vi "Main.vi"(0 "User Signal":u16 format="%.0x", 1 "Signal Operator":T1, 2 "Generate":bool, 5 "Speed Mode":T3, 7 "Target Address":u16 max=127 format="%.0x", 9 "Addressing bit":T2, 11 "Error In":errorcluster) -> (4 "Digital Waveform Graph":digitaldata(graph), 15 "Error out":errorcluster)   [LabVIEW 2020, in "I2C Controller.lvlib"]
doc: "This VI is to move from one state to other to perform ertain functionality."
uses:
  I2C Controller.lvlib
  Typedefs/Speed Control.ctl
  Typedefs/Addressing Bit.ctl
  Typedefs/Signal Operator.ctl
  Typedefs/Operator.ctl
  Typedefs/Controller Data.ctl
  Class/Parent Class/Speed Mode/Speed Mode.lvclass
  Class/Parent Class/Address/Address.lvclass
  Typedefs/User event operator.ctl
  <vilib>/numeric/Random Number (Range) U64.vi
  <vilib>/numeric/sub_Random U32.vi
panel:
  out "Read Signal":u64
  # "I2C Controller"
  # "Bit timing Parameters"
  # "Data"
  # "Generate signals"
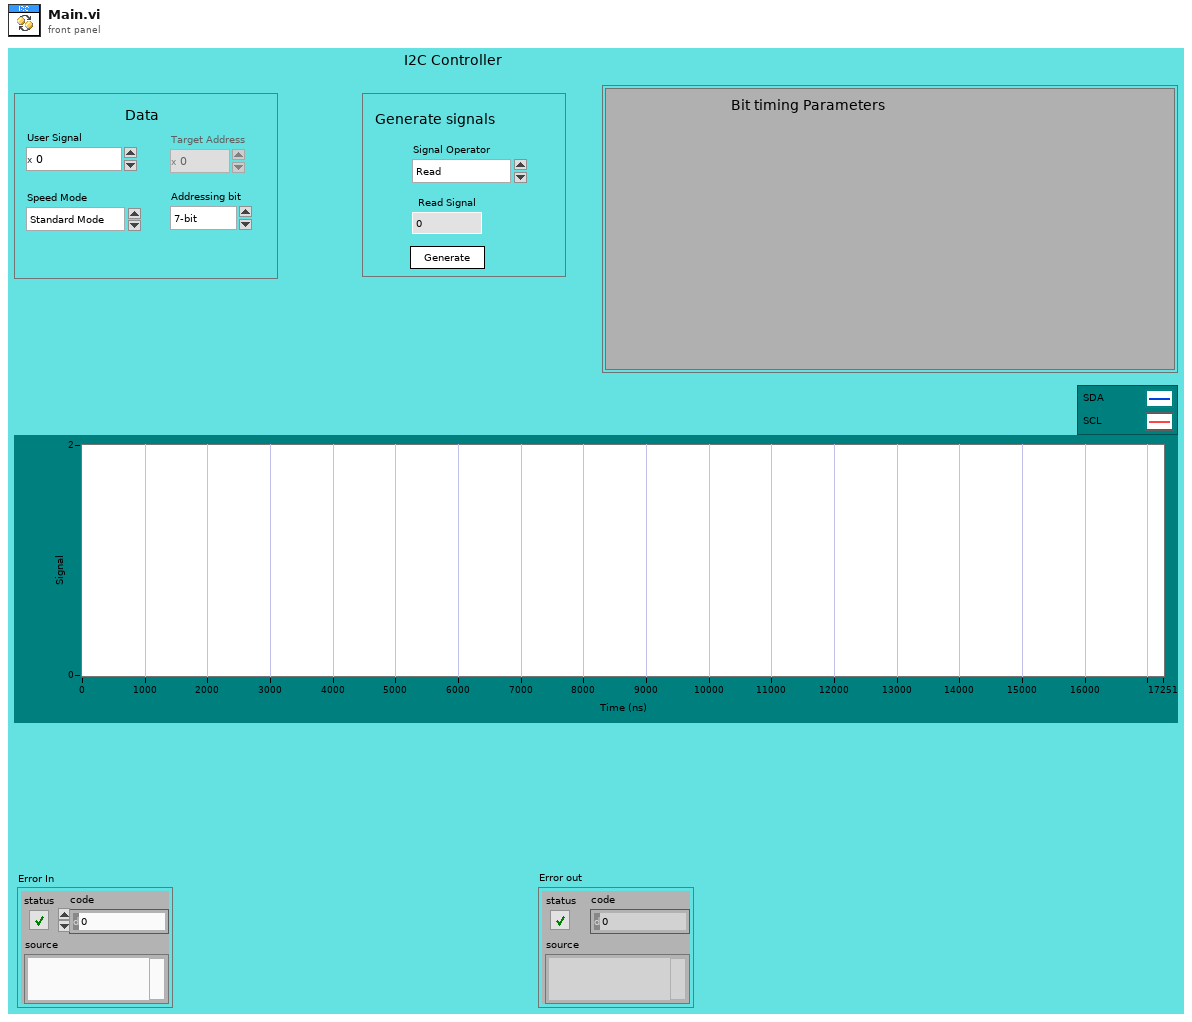
[diagram p1: front panel]
types:
  T1 = typedef "I2C Controller.lvlib/Signal Operator.ctl" = enum16{"Read", "Write", "Write-Read"}
  T2 = typedef "I2C Controller.lvlib/Addressing Bit.ctl" = enum16{"7-bit", "10-bit"}
  T3 = typedef "I2C Controller.lvlib/Speed Control.ctl" = enum16{"Standard Mode", "Fast Mode", "Fast-Plus Mode"}
  T4 = typedef "I2C Controller.lvlib/Controller Data.ctl" = cluster{"Target Address":u16, "User Signal":u8, "Read Signal":u64, "R/W Bit":i32, "Address Flag":bool, "Signal Size":i32, "Class Path":path, "Addressing bit":T2, "Speed Mode":T3, "Signal Operator":T1, "Generated Address":i16[], "User signal array":i16[], "Signal array":i16[], "Clock Signal":i16[], "Data":u8[][], "Time array":dbl[], "DVR Out":refnum<data-value>, "Addrerss DVR":refnum<data-value>, "Asynch Ref":refnum<vi>, "Digital Waveform Graph":digitaldata}
  T5 = typedef "I2C Controller.lvlib/Operator.ctl" = enum16{"Create Queue", "Enqueue", "Enstack", "Dequeue", "Flush Queue", "Release Queue"}
  T6 = typedef "I2C Controller.lvlib/User event operator.ctl" = enum16{"Create", "Generate Stop", "Destroy"}
  T7 = enum8{"Enabled", "Disabled", "Disabled and Grayed Out"}
  T8 = cluster{"Clock frequency":dbl, " T hd;sta":dbl, "T low":dbl, "T high":dbl, "T su;sta":dbl, "T hd;dat":dbl, "T su;dat":dbl, "T su;sto":dbl, "T buf":dbl}
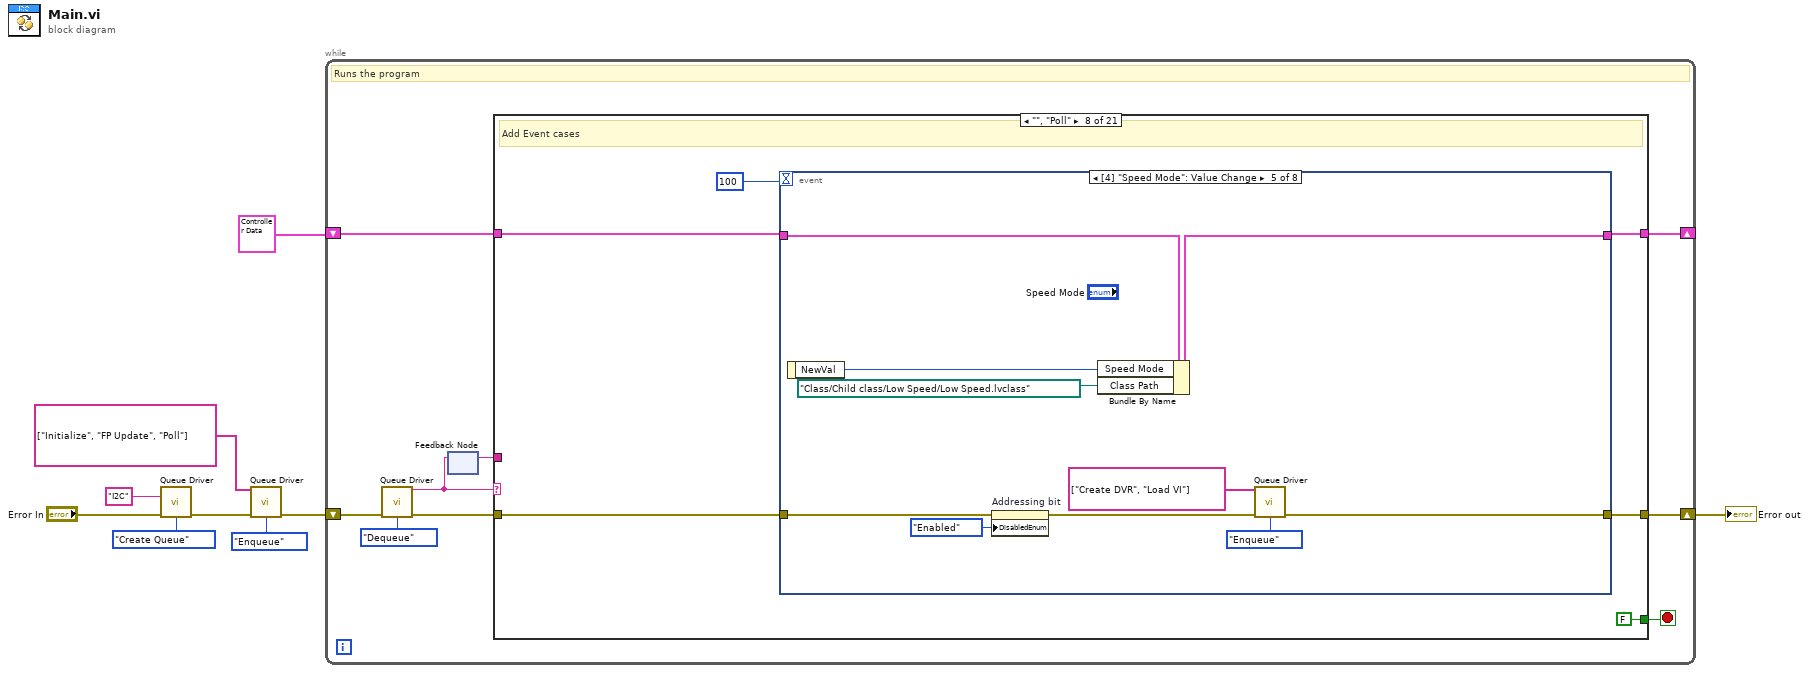
[diagram p0: block diagram]
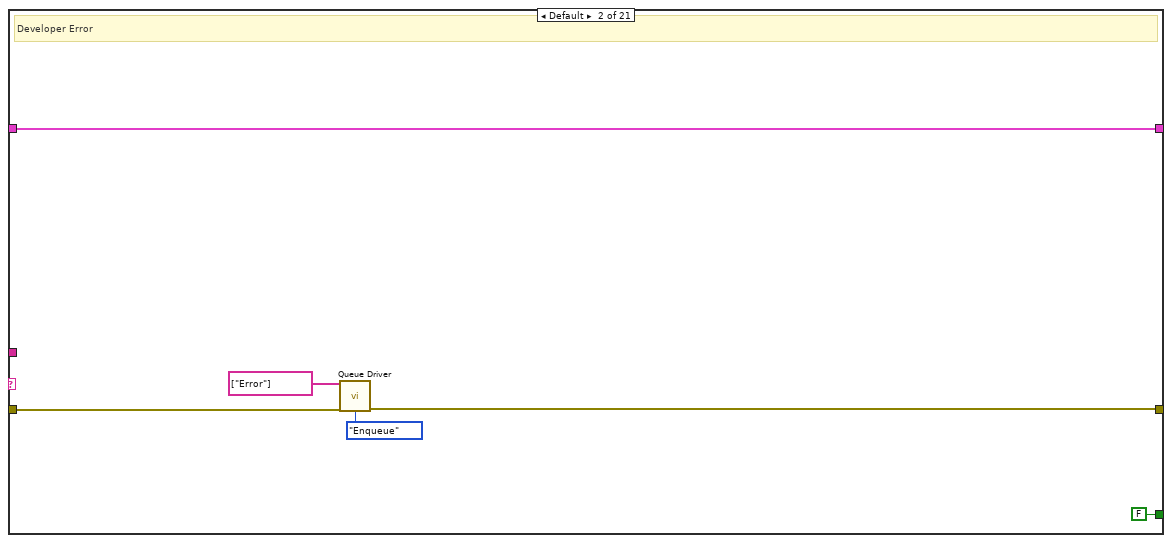
[diagram p3: hidden frame]
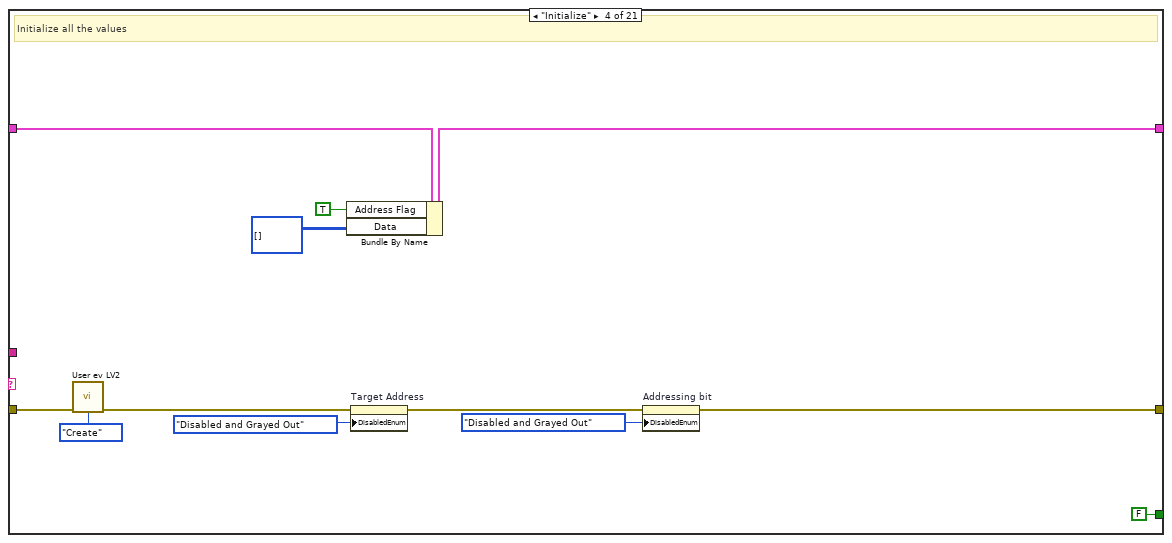
[diagram p5: hidden frame]
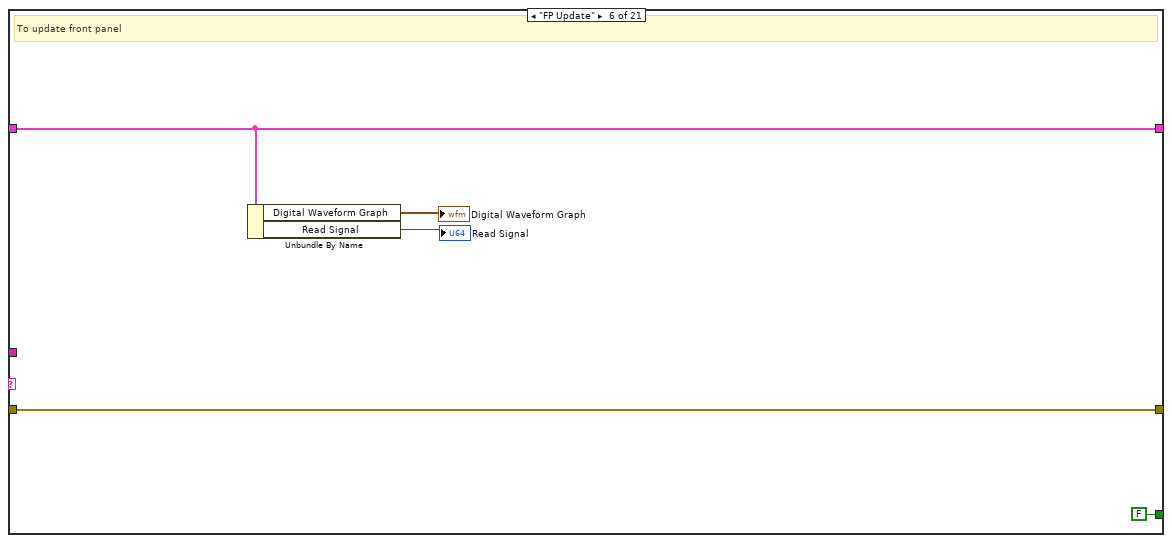
[diagram p7: hidden frame]
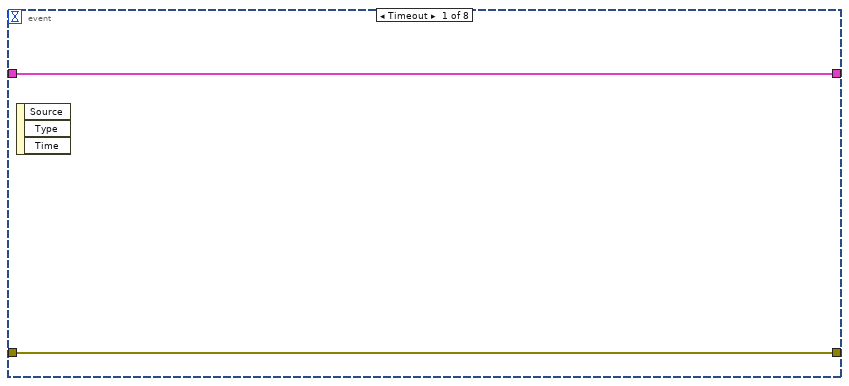
[diagram p9: hidden frame]
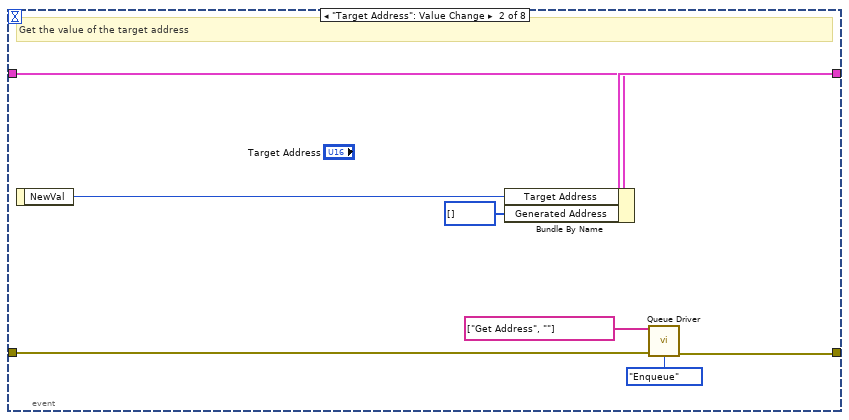
[diagram p10: hidden frame]
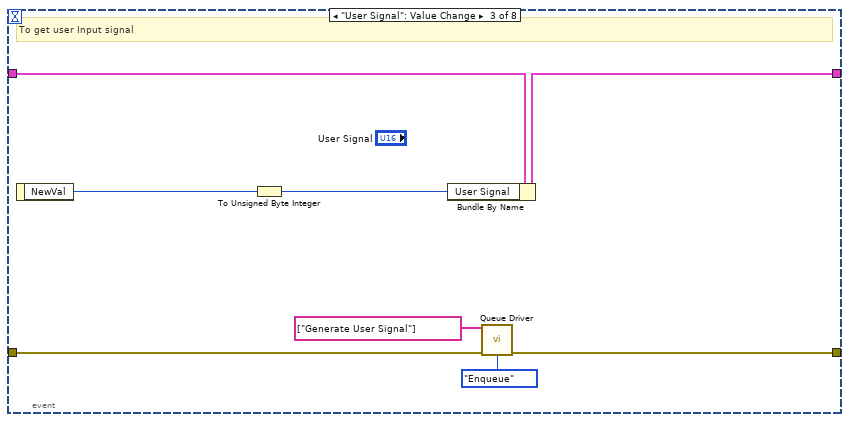
[diagram p11: hidden frame]
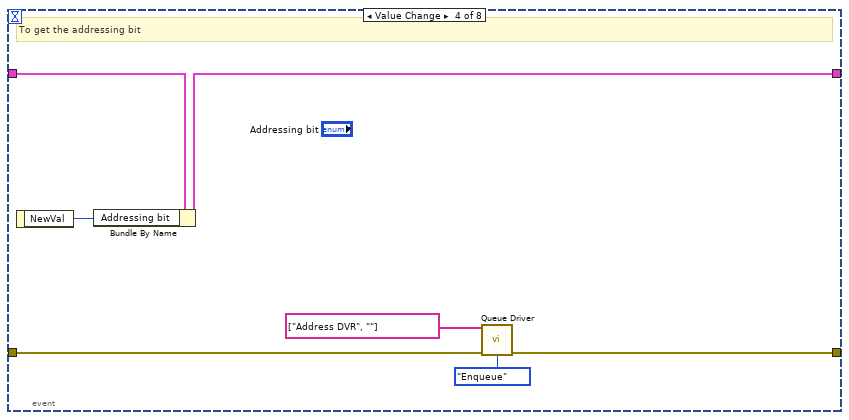
[diagram p12: hidden frame]
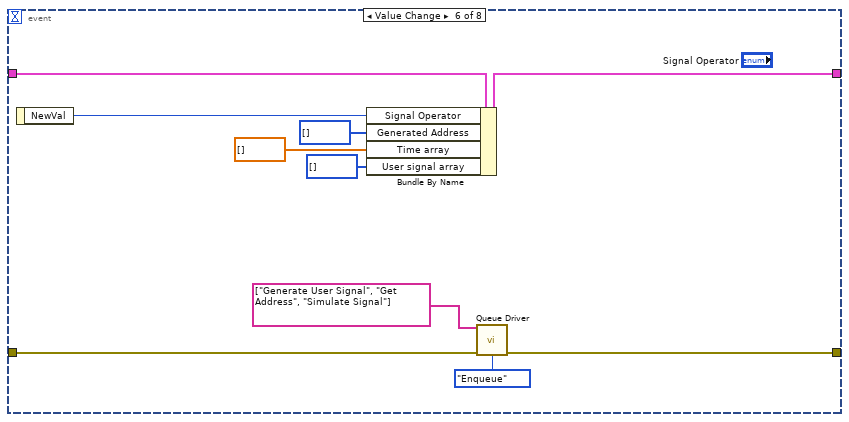
[diagram p13: hidden frame]
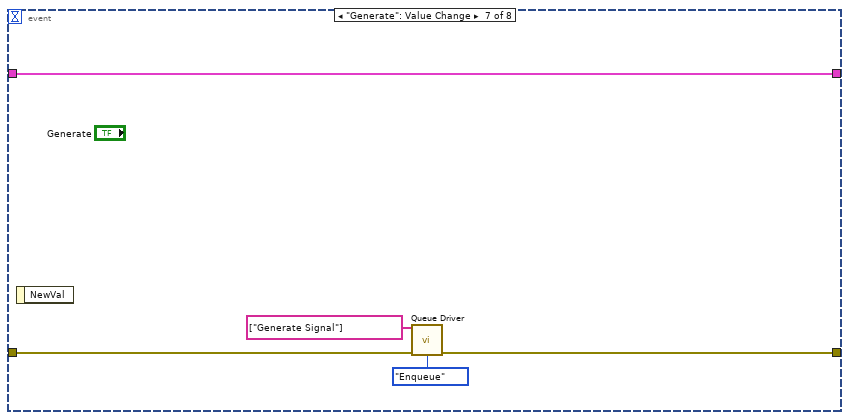
[diagram p14: hidden frame]
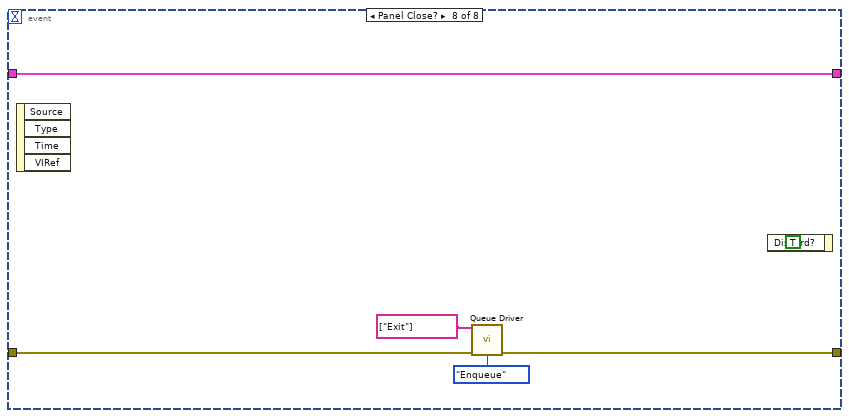
[diagram p15: hidden frame]
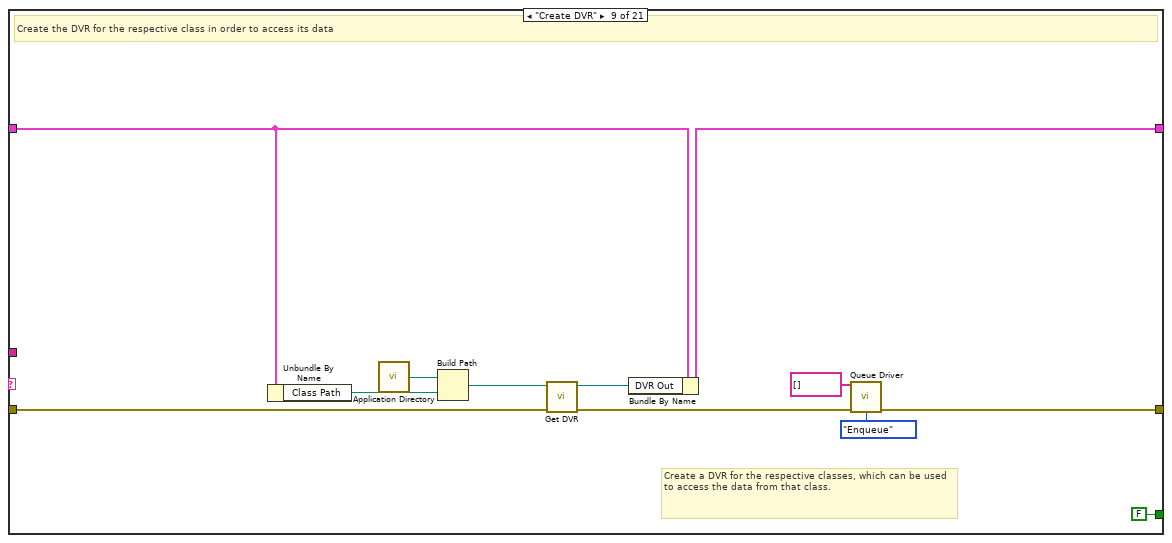
[diagram p16: hidden frame]
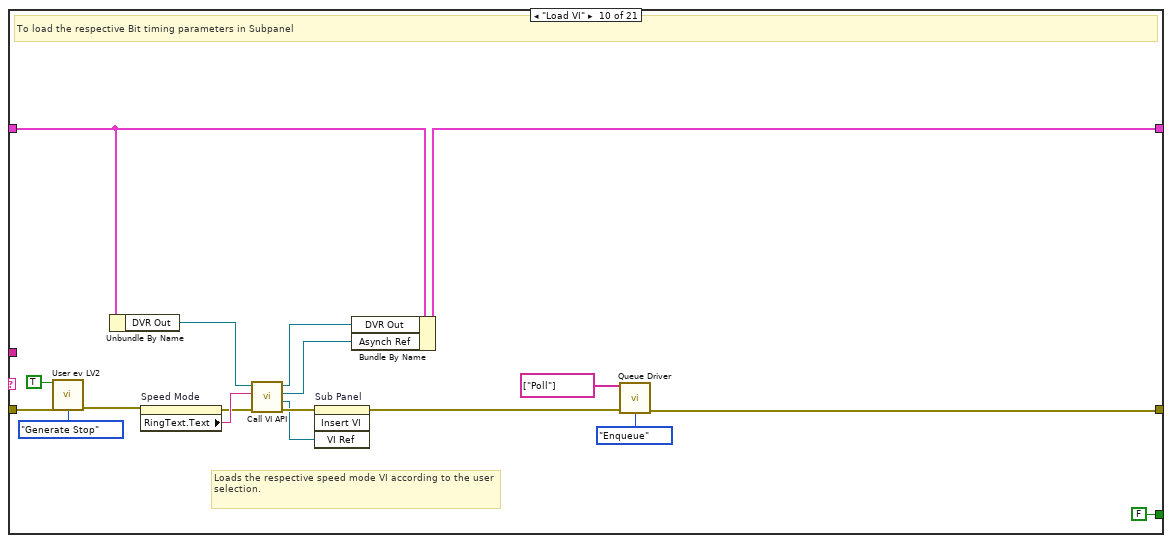
[diagram p17: hidden frame]
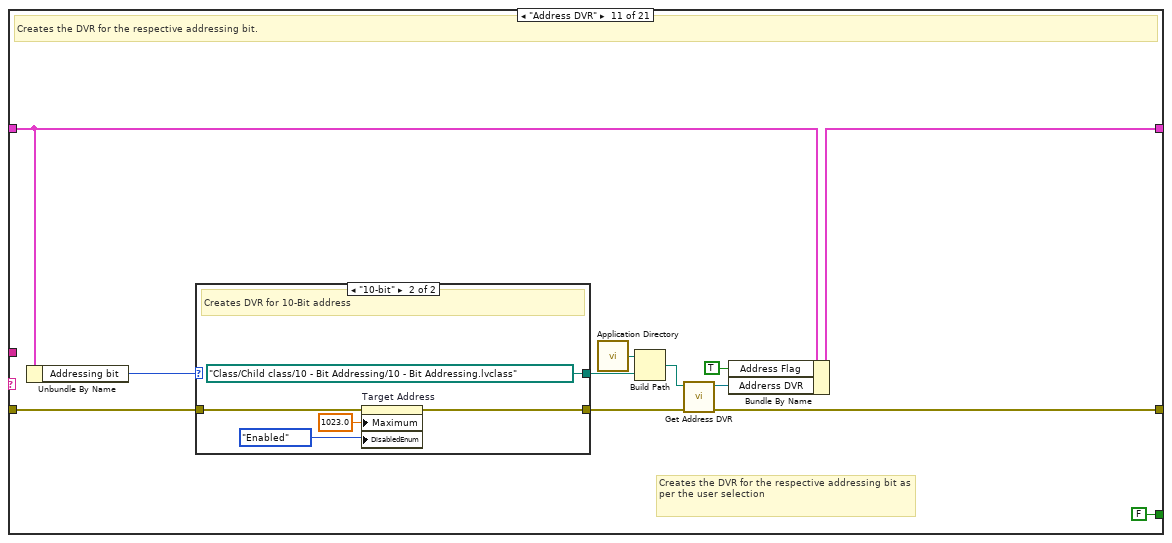
[diagram p18: hidden frame]
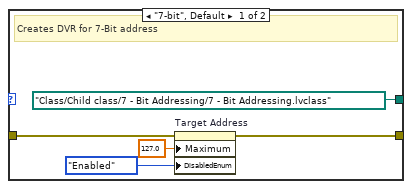
[diagram p19: hidden frame]
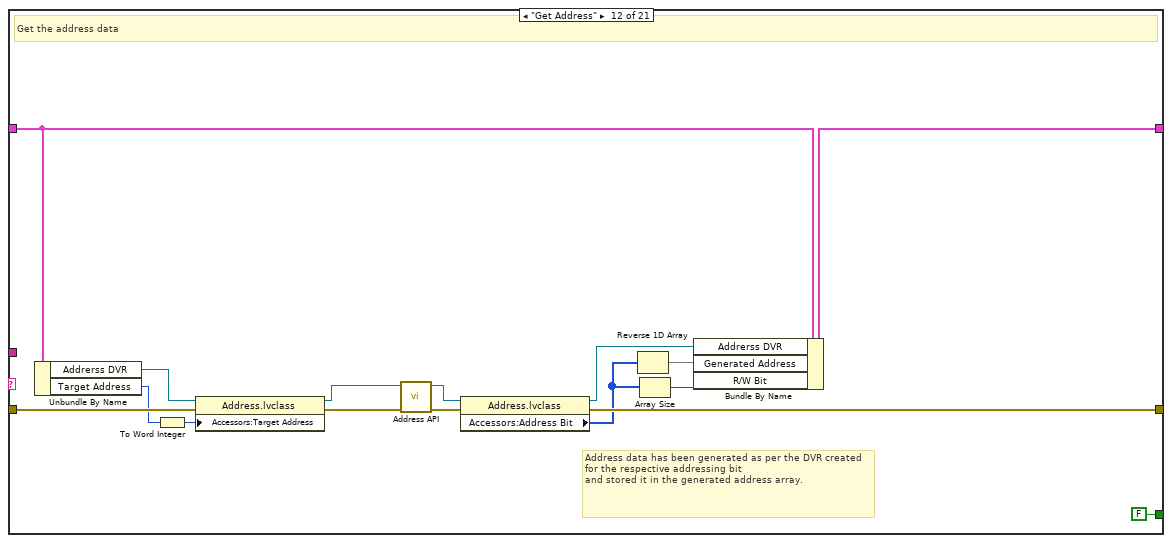
[diagram p20: hidden frame]
diagram:
  n1 = call "Queue Driver.vi"("Name"="I2C", "Error In"="Error In", "Operator"=Operator."Create Queue") -> ("Error out"=w9:errorcluster)  [unwired: 10 in, 2 out]
  n2 = call "Queue Driver.vi"("States []"=string[] ["Initialize", "FP Update", "Poll"], "Error In"=w9, "Operator"=Operator."Enqueue") -> ("Error out"=w3:errorcluster)  [unwired: 10 in, 2 out]
  n3 = while {
    shift-right: [w10] -> _
    shift-left: T4 {"Target Address"=0, "User Signal"=0, "Read Signal"=0, "R/W Bit"=0, "Address Flag"=FALSE, "Signal Size"=0, "Class Path"=path "", "Addressing bit"=enum."7-bit", "Speed Mode"=enum."Standard Mode", "Signal Operator"=enum."Read", "Generated Address"=[], "User signal array"=[], "Signal array"=[], "Clock Signal"=[], "Data"=[], "Time array"=[], "DVR Out"=refnum, "Addrerss DVR"=refnum, "Asynch Ref"=refnum, "Digital Waveform Graph"={"transitions"=[], "data"=[]}} -> [w11]
    shift-right: [w14] -> w2
    shift-left: w3 -> [w18]
    stop <- w15 stop-if-true
    # "Runs the program"
    n4 = call "Queue Driver.vi"("Error In"=w18, "Operator"=Operator."Dequeue") -> ("Dequeued State"=w13:string, "Error out"=w16:errorcluster)  [unwired: 11 in, 1 out]
    n5 = feedback #1() -> (w12:string)  [unwired: 1 in]
    n6 = feedback-in #1(w13) -> ()
    n7 = case shown="\"\", \"Poll\"" w13 {
      tunnel: w16 -> [w20 w26 w28 w40 w42 w45 w49 w55 w123 w130 w145 w179 w187 w199 w245 w267 w308 w324 w330 w333 w336]
      tunnel: [_ FALSE _ FALSE _ FALSE _ FALSE FALSE FALSE FALSE FALSE FALSE FALSE FALSE FALSE FALSE _ TRUE _ FALSE] -> w15
      tunnel: [w20 w25 w28 w37 w42 w45 w49 w53 w114 w141 w149 w177 w187 w193 w242 w266 w316 w324 w326 w333 w350] -> w14
      tunnel: w12 -> [_ _ _ _ _ _ _ _ _ _ _ _ _ _ _ _ _ _ _ _ w342]
      tunnel: w11 -> [w19 w22 w27 w33 w41 w47 w48 w51 w118 w138 w151 w170 w183 w197 w239 w263 w318 w323 w325 w332 w337]
      tunnel: [w19 w22 w27 w31 w41 w47 w48 w52 w119 w137 w150 w168 w181 w196 w238 w262 w317 w323 w325 w332 w337] -> w10
      frame "**********Default**********" {
        # "Splitter"
      }
      frame Default {
        # "Developer Error"
        n8 = call "Queue Driver.vi"("States []"=string[] ["Error"], "Error In"=w26, "Operator"=Operator."Enqueue") -> ("Error out"=w25:errorcluster)  [unwired: 10 in, 2 out]
      }
      frame "**********Initialize**********" {
        # "Splitter"
      }
      frame "Initialize" {
        # "Initialize all the values"
        n9 = call "User ev LV2.vi"("Error in"=w40, "User Event Operator"=User_event_operator."Create") -> ("Error out"=w35:errorcluster)  [unwired: 12 in, 1 out]
        n10 = Bundle By Name(cluster=w33, "Address Flag"=TRUE, "Data"=u8[][] []) -> (w31:T4)
        n11 = property on="Target Address" class="DigNum (strict)"(error in=w35, "DisabledEnum"=T7."Disabled and Grayed Out" ("Disabled")) -> (error out=w39:errorcluster)  [unwired: 1 in, 1 out]
        n12 = property on="Addressing bit" class="Enum (strict)"(error in=w39, "DisabledEnum"=T7."Disabled and Grayed Out" ("Disabled")) -> (error out=w37:errorcluster)  [unwired: 1 in, 1 out]
      }
      frame "**********FP Update**********" {
        # "Splitter"
      }
      frame "FP Update" {
        # "To update front panel"
        n13 = Unbundle By Name(w47) -> ("Digital Waveform Graph"=→"Digital Waveform Graph":digitaldata, "Read Signal"=→"Read Signal":u64)
      }
      frame "**********Functionality**********" {
        # "Splitter"
      }
      frame "", "Poll" {
        # "Add Event cases"
        n14 = event shown="[4] \"Speed Mode\": Value Change" {
          selector: _ -> [_ _ _ _ _ _ _ _]
          dyn-events: _ -> [_ _ _ _ _ _ _ _]
          timeout: 100 -> [_ _ _ _ _ _ _ _]
          tunnel: w55 -> [w57 w64 w73 w80 w90 w100 w105 w110]
          tunnel: [w57 w61 w69 w77 w81 w96 w104 w109] -> w53
          tunnel: [w56 w65 w70 w78 w87 w97 w101 w107] -> w52
          tunnel: w51 -> [w56 w62 w72 w79 w89 w99 w101 w107]
          event Timeout {
            n15 = event-data() -> ()  [unwired: 1 in, 3 out]
          }
          event "Target Address": Value Change {
            # "Get the value of the target address"
            n16 = event-data() -> ("NewVal"=w63:u16)  [unwired: 1 in]
            n17 = Bundle By Name(cluster=w62, "Target Address"=w63, "Generated Address"=i16[] []) -> (w65:T4)
            n18 = call "Queue Driver.vi"("States []"=string[] ["Get Address", ""], "Error In"=w64, "Operator"=Operator."Enqueue") -> ("Error out"=w61:errorcluster)  [unwired: 10 in, 2 out]
          }
          event "User Signal": Value Change {
            # "To get user Input signal"
            n19 = event-data() -> ("NewVal"=w71:u16)  [unwired: 1 in]
            n20 = To Unsigned Byte Integer(number=w71) -> (unsigned 8bit integer=w66:u8)
            n21 = Bundle By Name(cluster=w72, "User Signal"=w66) -> (w70:T4)
            n22 = call "Queue Driver.vi"("States []"=string[] ["Generate User Signal"], "Error In"=w73, "Operator"=Operator."Enqueue") -> ("Error out"=w69:errorcluster)  [unwired: 10 in, 2 out]
          }
          event Value Change {
            # "To get the addressing bit"
            n23 = event-data() -> ("NewVal"=w74:T2)  [unwired: 1 in]
            n24 = Bundle By Name(cluster=w79, "Addressing bit"=w74) -> (w78:T4)
            n25 = call "Queue Driver.vi"("States []"=string[] ["Address DVR", ""], "Error In"=w80, "Operator"=Operator."Enqueue") -> ("Error out"=w77:errorcluster)  [unwired: 10 in, 2 out]
          }
          event Value Change {
            n26 = event-data() -> ("NewVal"=w88:T3)  [unwired: 1 in]
            n27 = property on="Addressing bit" class="Enum (strict)"(error in=w90, "DisabledEnum"=T7."Enabled" ("Disabled")) -> (error out=w82:errorcluster)  [unwired: 1 in, 1 out]
            n28 = Bundle By Name(cluster=w89, "Speed Mode"=w88, "Class Path"=path "Class/Child class/Low Speed/Low Speed.lvclass") -> (w87:T4)
            n29 = call "Queue Driver.vi"("States []"=string[] ["Create DVR", "Load VI"], "Error In"=w82, "Operator"=Operator."Enqueue") -> ("Error out"=w81:errorcluster)  [unwired: 10 in, 2 out]
          }
          event Value Change {
            n30 = event-data() -> ("NewVal"=w98:T1)  [unwired: 1 in]
            n31 = Bundle By Name(cluster=w99, "Signal Operator"=w98, "Generated Address"=i16[] [], "Time array"=dbl[] [], "User signal array"=i16[] []) -> (w97:T4)
            n32 = call "Queue Driver.vi"("States []"=string[] ["Generate User Signal", "Get Address", "Simulate Signal"], "Error In"=w100, "Operator"=Operator."Enqueue") -> ("Error out"=w96:errorcluster)  [unwired: 10 in, 2 out]
          }
          event "Generate": Value Change {
            n33 = event-data() -> ()  [unwired: 1 in, 1 out]
            n34 = call "Queue Driver.vi"("States []"=string[] ["Generate Signal"], "Error In"=w105, "Operator"=Operator."Enqueue") -> ("Error out"=w104:errorcluster)  [unwired: 10 in, 2 out]
          }
          event Panel Close? {
            n35 = event-data() -> ()  [unwired: 1 in, 4 out]
            n36 = call "Queue Driver.vi"("States []"=string[] ["Exit"], "Error In"=w110, "Operator"=Operator."Enqueue") -> ("Error out"=w109:errorcluster)  [unwired: 10 in, 2 out]
            n37 = event-data("Discard?"=TRUE) -> ()  [unwired: 1 in, 1 out]
          }
        }
      }
      frame "Create DVR" {
        # "Create a DVR for the respective classes, which can be used to access the data from that class."
        # "Create the DVR for the respective class in order to access its data"
        n38 = Unbundle By Name(w118) -> ("Class Path"=w117:path)
        n39 = call <vilib>:"Application Directory.vi"() -> ("Application Directory"=w121:path)
        n40 = Build Path(base path=w121, name or relative path=w117) -> (appended path=w120:path)
        n41 = call "Get DVR.vi"("Error in"=w123, "class path"=w120) -> ("Error out"=w122:errorcluster, "DVR Out"=w116:refnum<data-value>)  [unwired: 8 in]
        n42 = Bundle By Name(cluster=w118, "DVR Out"=w116) -> (w119:T4)
        n43 = call "Queue Driver.vi"("States []"=string[] [], "Error In"=w122, "Operator"=Operator."Enqueue") -> ("Error out"=w114:errorcluster)  [unwired: 10 in, 2 out]
      }
      frame "Load VI" {
        # "Loads the respective speed mode VI according to the user selection."
        # "To load the respective Bit timing parameters in Subpanel"
        n44 = call "User ev LV2.vi"("Stop"=TRUE, "Error in"=w130, "User Event Operator"=User_event_operator."Generate Stop") -> ("Error out"=w129:errorcluster)  [unwired: 11 in, 1 out]
        n45 = Unbundle By Name(w138) -> ("DVR Out"=w136:refnum<data-value>)
        n46 = property on="Speed Mode" class="Enum (strict)"(error in=w129) -> (error out=w134:errorcluster, "RingText.Text"=w135:string)  [unwired: 1 in, 1 out]
        n47 = call "Call VI API.vi"("error in"=w134, "Section"=w135, "DVR In"=w136) -> ("error out"=w133:errorcluster, "VI Ref"=w132:refnum<vi>, "Asynch Ref"=w125:refnum<vi>, "DVR Out"=w127:refnum<data-value>)  [unwired: 5 in]
        n48 = invoke on="Sub Panel" class="SubPnl" method="Insert VI"(error in=w133, "VI Ref"=w132) -> (error out=w128:errorcluster)  [unwired: 2 in, 3 out]
        n49 = Bundle By Name(cluster=w138, "DVR Out"=w127, "Asynch Ref"=w125) -> (w137:T4)
        n50 = call "Queue Driver.vi"("States []"=string[] ["Poll"], "Error In"=w128, "Operator"=Operator."Enqueue") -> ("Error out"=w141:errorcluster)  [unwired: 10 in, 2 out]
      }
      frame "Address DVR" {
        # "Creates the DVR for the respective addressing bit as per the user selection"
        # "Creates the DVR for the respective addressing bit."
        n51 = Unbundle By Name(w151) -> ("Addressing bit"=w147:T2)
        n52 = case shown="\"10-bit\"" w147 {
          tunnel: [path "Class/Child class/7 - Bit Addressing/7 - Bit Addressing.lvclass" path "Class/Child class/10 - Bit Addressing/10 - Bit Addressing.lvclass"] -> w146
          tunnel: [w156 w161] -> w144
          tunnel: w145 -> [w157 w162]
          frame "7-bit", Default {
            # "Creates DVR for 7-Bit address"
            n53 = property on="Target Address" class="DigNum (strict)"(error in=w157, "Maximum"=127.0 ("Data Entry Limits:Maximum"), "DisabledEnum"=T7."Enabled" ("Disabled")) -> (error out=w156:errorcluster)  [unwired: 1 in, 1 out]
          }
          frame "10-bit" {
            # "Creates DVR for 10-Bit address"
            n54 = property on="Target Address" class="DigNum (strict)"(error in=w162, "Maximum"=1023.0 ("Data Entry Limits:Maximum"), "DisabledEnum"=T7."Enabled" ("Disabled")) -> (error out=w161:errorcluster)  [unwired: 1 in, 1 out]
          }
        }
        n55 = call <vilib>:"Application Directory.vi"() -> ("Application Directory"=w153:path)
        n56 = Build Path(base path=w153, name or relative path=w146) -> (appended path=w152:path)
        n57 = call "Get Address DVR.vi"("error in"=w144, "class path"=w152) -> ("error out"=w149:errorcluster, "DVR Out"=w148:refnum<data-value>)  [unwired: 8 in]
        n58 = Bundle By Name(cluster=w151, "Address Flag"=TRUE, "Addrerss DVR"=w148) -> (w150:T4)
      }
      frame "Get Address" {
        # "Address data has been generated as per the DVR created for the respective addressing bit\nand stored it in the generated address array."
        # "Get the address data"
        n59 = Unbundle By Name(w170) -> ("Addrerss DVR"=w174:refnum<data-value>, "Target Address"=w172:u16)
        n60 = To Word Integer(number=w172) -> (16bit integer=w171:i16)
        n61 = property class="Address.lvclass"(reference=w174, error in=w179, "Accessors:Target Address"=w171) -> (reference out=w173:refnum<data-value>, error out=w175:errorcluster)
        n62 = call "Address API.vi"("error in"=w175, "DVR"=w173) -> ("error out"=w178:errorcluster, "DVR Out"=w176:refnum<data-value>)  [unwired: 8 in]
        n63 = property class="Address.lvclass"(reference=w176, error in=w178) -> (reference out=w169:refnum<data-value>, error out=w177:errorcluster, "Accessors:Address Bit"=w167:i16[])
        n64 = Reverse 1D Array(array=w167) -> (reversed array=w165:i16[])
        n65 = Array Size(array=w167) -> (size(s)=w166:i32)
        n66 = Bundle By Name(cluster=w170, "Addrerss DVR"=w169, "Generated Address"=w165, "R/W Bit"=w166) -> (w168:T4)
      }
      frame "Generate User Signal" {
        # "Generate User Signal array"
        n67 = Unbundle By Name(w183) -> ("User Signal"=w186:u8)
        n68 = Number To Boolean Array(number=w186) -> (Boolean array=w185:bool[])
        n69 = Boolean To (0,1)(Boolean=w185) -> (0, 1=w184:i16[])
        n70 = Reverse 1D Array(array=w184) -> (reversed array=w182:i16[])
        n71 = Bundle By Name(cluster=w183, "User signal array"=w182) -> (w181:T4)
      }
      frame "Simulate Signal" {
        # "Add the read/write to the gene"
        n72 = Unbundle By Name(w197) -> ("R/W Bit"=w189:i32, "Signal Operator"=w200:T1, "Generated Address"=w195:i16[])
        n73 = case shown="\"Write\", Default" w200 {
          tunnel: w199 -> [w208 w214 w225]
          tunnel: [w208 w214 w225] -> w198
          tunnel: w195 -> [w201 w213 w224]
          tunnel: [w204 w210 w220] -> w194
          tunnel: [w205 u64 0 ("number") w217] -> w190
          tunnel: w189 -> [w202 w209 w216]
          frame "Read" {
            # "Generate read bit"
            n74 = call-poly <vilib>:"Random Number (Range).vi"("lower bound (0)"=u64 0, "upper bound (100)"=u64 127) -> ("number"=w205:u64)  [unwired: 9 in]
            n75 = Insert Into Array(array=w201, index=w202, new element=i16 1 ("new element/subarray")) -> (w204:i16[])
          }
          frame "Write", Default {
            # "Generate write bit"
            n76 = Insert Into Array(array=w213, index=w209, new element=i16 0 ("new element/subarray")) -> (w210:i16[])
          }
          frame "Write-Read" {
            # "Generate read write bit"
            n77 = Insert Into Array(array=w224, index=w216, new element=i16 0 ("new element/subarray")) -> (w222:i16[])
            n78 = Increment(x=w216) -> (x+1=w215:i32)
            n79 = call-poly <vilib>:"Random Number (Range).vi"("lower bound (0)"=u64 0, "upper bound (100)"=u64 127) -> ("number"=w217:u64)  [unwired: 9 in]
            n80 = Insert Into Array(array=w222, index=w215, new element=i16 1 ("new element/subarray")) -> (w220:i16[])
          }
        }
        n81 = call "Queue Driver.vi"("States []"=string[] ["Signal", ""], "Error In"=w198, "Operator"=Operator."Enqueue") -> ("Error out"=w193:errorcluster)  [unwired: 10 in, 2 out]
        n82 = Bundle By Name(cluster=w197, "Read Signal"=w190, "Generated Address"=w194) -> (w196:T4)
      }
      frame "Signal" {
        # "Stop bit"
        # "Ack Bit"
        # "start bit"
        # "Generate signal array with all the necessary bit."
        n83 = Unbundle By Name(w239) -> ("User signal array"=w243:i16[], "Generated Address"=w234:i16[], "Address Flag"=w235:bool, "R/W Bit"=w236:i32)
        n84 = Increment(x=w236) -> (x+1=w237:i32)
        n85 = case shown="False" w235 {
          tunnel: w234 -> [w246 w248]
          tunnel: [w246 w247] -> w233
          frame False {
          }
          frame True {
            n86 = Insert Into Array(array=w248, index=0, new element=i16 1 ("new element/subarray")) -> (w247:i16[])
          }
        }
        n87 = Insert Into Array(array=w233, index=w237, new element=i16 1 ("new element/subarray")) -> (w232:i16[])
        n88 = Insert Into Array(array=w232, new element=w243) -> (w230:i16[])  [unwired: 1 in]
        n89 = Insert Into Array(array=w230, new element=w230) -> (w229:i16[])  [unwired: 1 in]
        n90 = call "Queue Driver.vi"("States []"=string[] ["Generate Time"], "Error In"=w245, "Operator"=Operator."Enqueue") -> ("Error out"=w242:errorcluster)  [unwired: 10 in, 2 out]
        n91 = Insert Into Array(array=w229, new element=i16 0 ("new element/subarray")) -> (w228:i16[])  [unwired: 1 in]
        n92 = Array Size(array=w228) -> (size(s)=w227:i32)
        n93 = Bundle By Name(cluster=w239, "Signal Size"=w227, "Signal array"=w228, "Generated Address"=w233) -> (w238:T4)
      }
      frame "Generate Time" {
        # "Time array is getting generated according to which the data transition has to happen."
        # "To get Time array for transition"
        n94 = Unbundle By Name(w263) -> ("Signal array"=w257:i16[], "Time array"=w256:dbl[], "DVR Out"=w255:refnum<data-value>)
        n95 = Array Size(array=w257) -> (size(s)=w251:i32)
        n96 = property class="Speed Mode.lvclass"(reference=w255, error in=w267) -> (reference out=w253:refnum<data-value>, error out=w266:errorcluster, "Accessors:Time parameter"=w265:T8)
        n97 = Unbundle By Name(w265) -> ("T low"=w259:dbl, "T high"=w264:dbl, "T hd;sta"=w258:dbl, "T su;sto"=w254:dbl)
        n98 = for {
          tunnel: w257 -> [w271] mode=indexing
          tunnel: w264 -> [w269]
          shift-right: [w272] -> w260
          shift-left: w256 -> [w274]
          tunnel: w258 -> [w273]
          tunnel: w259 -> [w270]
          tunnel: w254 -> [w268]
          i -> [w275]
          # "To generate Time array for transitionf of data"
          n99 = Equal To 0?(x=w275) -> (x = 0?=w276:bool)
          n100 = case shown="True" w276 {
            tunnel: w274 -> [w279 w289]
            tunnel: w273 -> [_ w293]
            tunnel: [w278 w291] -> w272
            tunnel: w271 -> [w282 _]
            tunnel: w270 -> [w281 _]
            tunnel: w269 -> [w280 _]
            tunnel: w268 -> [_ _]
            frame False {
              # "To get time for subsequent data signal"
              n101 = Array Size(array=w279) -> (size(s)=w285:i32)
              n102 = Decrement(x=w285) -> (x-1=w284:i32)
              n103 = Equal To 0?(x=w282) -> (x = 0?=w287:bool)
              n104 = Index Array(array=w279, index=w284) -> (element=w283:dbl)
              n105 = Select(t=w281, s=w287, f=w280) -> (s? t:f=w286:dbl)
              n106 = Add(x=w286, y=w283) -> (x+y=w277:dbl)
              n107 = Insert Into Array(array=w279, new element=w277) -> (w278:dbl[])  [unwired: 1 in]
            }
            frame True {
              # "To get time for start bit signal data"
              n108 = Array Size(array=w289) -> (size(s)=w295:i32)
              n109 = Decrement(x=w295) -> (x-1=w296:i32)
              n110 = Equal To 0?(x=w295) -> (x = 0?=w297:bool)
              n111 = Select(t=w295, s=w297, f=w296) -> (s? t:f=w294:i32)
              n112 = Index Array(array=w289, index=w294) -> (element=w288:dbl)
              n113 = Add(x=w288, y=w293) -> (x+y=w290:dbl)
              n114 = Insert Into Array(array=w289, index=0, new element=w290) -> (w291:dbl[])
            }
          }
        }
        n115 = Array Subset(array=w260, length=w251) -> (w252:dbl[])  [unwired: 1 in]
        n116 = Bundle By Name(cluster=w263, "Signal Size"=w251, "Time array"=w252, "DVR Out"=w253) -> (w262:T4)
      }
      frame "Generate Signal" {
        # "Generate graph data signal"
        n117 = Unbundle By Name(w318) -> ("Data"=w299:u8[][], "Signal Size"=w304:i32, "Signal array"=w305:i16[], "Time array"=w302:dbl[])
        n118 = for {
          N: w304 -> [_]
          tunnel: [w322] -> w306 mode=concatenating
          n119 = Insert Into Array(array=i32[] [] ("y"), new element #1=0 ("new element/subarray"), new element #2=1 ("new element/subarray")) -> (w322:i32[])  [unwired: 1 in]
        }
        n120 = To Unsigned Long Integer(number=w302) -> (unsigned 32bit integer=w307:u32[])
        n121 = To Word Integer(number=w306) -> (16bit integer=w303:i16[])
        n122 = Insert Into Array(array=i16[][] [], new element #1=w303, new element #2=w305) -> (w310:i16[][])  [unwired: 2 in]
        n123 = Transpose 2D Array(2D array=w310) -> (transposed array=w313:i16[][])
        n124 = call "Queue Driver.vi"("States []"=string[] ["FP Update"], "Error In"=w308, "Operator"=Operator."Enqueue") -> ("Error out"=w316:errorcluster)  [unwired: 10 in, 2 out]
        n125 = To Unsigned Byte Integer(number=w313) -> (unsigned 8bit integer=w300:u8[][])
        n126 = Insert Into Array(array=w299, new element=w300) -> (w301:u8[][])  [unwired: 2 in]
        n127 = Bundle By Name("data"=w301, "transitions"=w307) -> (w312:digitaldata)  [unwired: 1 in]
        n128 = Bundle By Name(cluster=w318, "Clock Signal"=w303, "Digital Waveform Graph"=w312, "Address Flag"=FALSE, "Data"=w301) -> (w317:T4)
      }
      frame "**********Exit**********" {
        # "Splitter"
      }
      frame "Exit" {
        # "To stop the program"
        n129 = call "Queue Driver.vi"("Error In"=w330, "Operator"=Operator."Flush Queue") -> ("Error out"=w327:errorcluster)  [unwired: 11 in, 2 out]
        n130 = call "Queue Driver.vi"("Error In"=w327, "Operator"=Operator."Release Queue") -> ("Error out"=w326:errorcluster)  [unwired: 11 in, 2 out]
      }
      frame "**********Error**********" {
        # "Splitter"
      }
      frame "Error" {
        # "To indentify the error that occured"
        n131 = Unbundle By Name(w336) -> ("code"=w335:i32, "source"=w353:string)
        n132 = call <vilib>:"Clear Errors.vi"("error in (no error)"=w336, "specific error code to clear (0: all)"=w335) -> ("error out"=w344:errorcluster)  [unwired: 4 in, 1 out]
        n133 = Format Into String(format string="Error State:  %s\n\nError Code : %d\n\nDescription: %s\n\nDo you want to continue?", error in=w344, w342, w335, w353) -> (resulting string=w339:string, error out=w355:errorcluster)  [unwired: 1 in]
        n134 = Equal?(x=w342, y="Default") -> (x = y?=w343:bool)
        n135 = Select(t="Developer Error" ("y"), s=w343, f=w339) -> (s? t:f=w338:string)
        n136 = Two Button Dialog(message=w338, 1:"No" ("T button name (\"OK\")"), 2:"Yes" ("T button name (\"OK\")")) -> (T button?=w349:bool)
        n137 = Select(t=string[] ["Poll"] ("T button name (\"OK\")"), s=w349, f=string[] ["Exit"] ("T button name (\"OK\")")) -> (s? t:f=w346:string[])
        n138 = call "Queue Driver.vi"("States []"=w346, "Error In"=w355, "Operator"=Operator."Enqueue") -> ("Error out"=w350:errorcluster)  [unwired: 10 in, 2 out]
      }
    }
  }
  "Error out" <- w2
